vi "CaseStatement.vi"() -> ()   [LabVIEW 2011]
panel:
  in  "Operation":enum16{"Add", "Subtract", "Multiply", "Divide"}(ring)
  out "Result":dbl
  in  "B":dbl
  in  "A":dbl
  out "Multiplied":bool
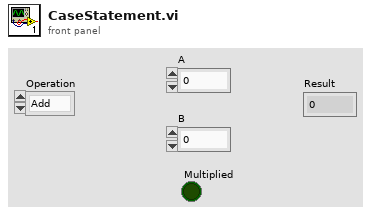
[diagram p1: front panel]
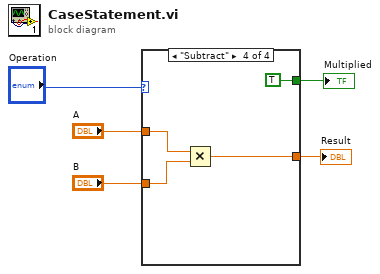
[diagram p0: block diagram]
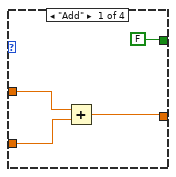
[diagram p2: hidden frame]
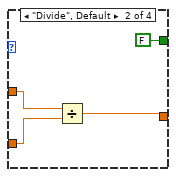
[diagram p3: hidden frame]
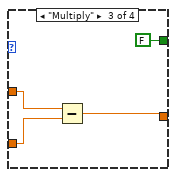
[diagram p4: hidden frame]
diagram:
  n1 = case shown="\"Subtract\"" "Operation" {
    tunnel: "A" -> [w9 w12 w16 w21]
    tunnel: "B" -> [w8 w11 w15 w20]
    tunnel: [w7 w10 w14 w19] -> w3
    tunnel: [FALSE FALSE FALSE TRUE] -> w2
    frame "Add" {
      n2 = Add(x=w9, y=w8) -> (x+y=w7:dbl)
    }
    frame "Divide", Default {
      n3 = Divide(x=w12, y=w11) -> (x/y=w10:dbl)
    }
    frame "Multiply" {
      n4 = Subtract(x=w16, y=w15) -> (x-y=w14:dbl)
    }
    frame "Subtract" {
      n5 = Multiply(x=w21, y=w20) -> (x*y=w19:dbl)
    }
  }
  "Multiplied" <- w2
  "Result" <- w3
